vi "gfitsio-change-endian.vi"(9 "word size (bytes)":i32, 11 "data in":u8[](array[numeric])) -> (3 "data out":u8[](array[numeric]))   [LabVIEW 2019, in "gfitsio.lvlib"]
uses:
  gfitsio.lvlib
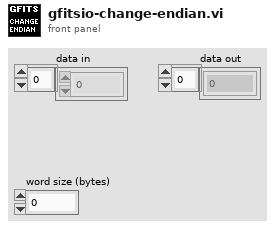
[diagram p1: front panel]
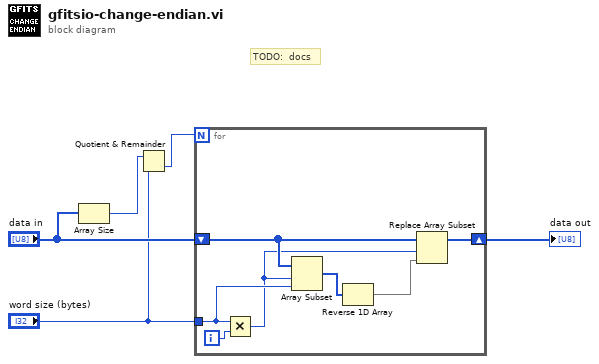
[diagram p0: block diagram]
diagram:
  # "TODO:  docs"
  n1 = Array Size(array="data in") -> (size(s)=w2:i32)
  n2 = Quotient & Remainder(x=w2, y="word size (bytes)") -> (floor(x/y)=w3:i32)  [unwired: 1 out]
  n3 = for {
    N: w3 -> [_]
    shift-right: [w11] -> w5
    shift-left: "data in" -> [w12]
    tunnel: "word size (bytes)" -> [w9]
    i -> [w10]
    n4 = Multiply(x=w9, y=w10) -> (x*y=w6:i32)
    n5 = Array Subset(array=w12, index=w6, length=w9) -> (w8:u8[])
    n6 = Reverse 1D Array(array=w8) -> (reversed array=w7:u8[])
    n7 = Replace Array Subset(array=w12, new element=w7, index=w6) -> (w11:u8[])
  }
  "data out" <- w5
